vi "saturatore_bipolare_progressivo.vi"(1 "waveform":waveform(dbl), 2 "V*":dbl min=0.0, 3 "Vfs":dbl min=0.0) -> (0 "output waveform":waveform(dbl))   [LabVIEW 2009]
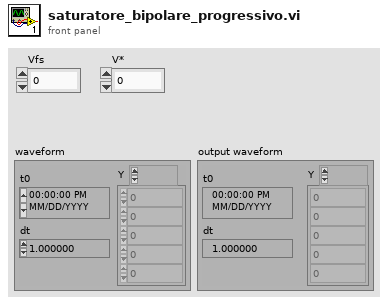
[diagram p1: front panel]
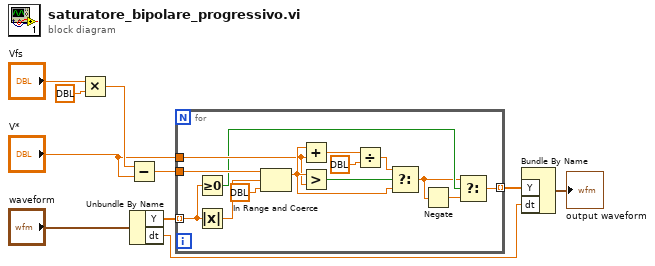
[diagram p0: block diagram]
diagram:
  n1 = Multiply(x="Vfs", y=dbl ?) -> (x*y=w5:dbl)
  n2 = Subtract(x=w5, y="V*") -> (x-y=w3:dbl)
  n3 = Unbundle By Name("waveform") -> ("Y"=w4:dbl[], "dt"=w9:dbl)
  n4 = for {
    tunnel: w4 -> [w24] mode=indexing
    tunnel: w3 -> [w21]
    tunnel: "V*" -> [w15]
    tunnel: [w11] -> w1 mode=indexing
    n5 = Greater Or Equal To 0?(x=w24) -> (x >= 0?=w14:bool)
    n6 = Absolute Value(x=w24) -> (abs(x)=w23:dbl)
    n7 = In Range and Coerce(upper limit=w21, x=w23, lower limit=dbl ?) -> (coerced(x)=w16:dbl)  [unwired: 1 out]
    n8 = Add(x=w16, y=w15) -> (x+y=w19:dbl)
    n9 = Greater?(x=w16, y=w15) -> (0:w18:bool)
    n10 = Divide(x=w19, y=dbl ?) -> (x/y=w20:dbl)
    n11 = Select(t=w20, s=w18, f=w16) -> (s? t:f=w13:dbl)
    n12 = Negate(x=w13) -> (-x=w12:dbl)
    n13 = Select(t=w13, s=w14, f=w12) -> (s? t:f=w11:dbl)
  }
  n14 = Bundle By Name("Y"=w1, "dt"=w9) -> (→"output waveform":waveform(dbl))  [unwired: 1 in]
